vi "config_TRIG1.vi"(10 "VISA resource name":refnum<visa-resource-name>="TRIG") -> ()   [LabVIEW 2011]
uses:
  global.vi
  <vilib>/Platform/browser.llb/Open URL in Default Browser (string).vi
panel:
  out "delay array":dbl[](array[numeric])=[0.0, 4.7525e-05, 0.0, 5.65e-06, 0.0, 5.65e-06, 7.5e-06, 4.75e-05, 7.3e-06, 1.23e-05]
  in  "duration":dbl[](array[numeric])=[47.525000000000006, 5.65, 5.65, 40.0, 5.0] min=0.0 format="%.3f"
  in  "start time":dbl[](array[numeric])=[0.0, 0.0, 0.0, 7.5, 7.300000000000001] format="%.3f"
  in  "time unit":enum16{"s", "ms", "us", "ns"}(ring)=enum."us"
  in  "Reset TRIG":bool
  in  "write config":bool
  in  "stop":bool
  in  "help":bool
  out "update front panel":bool
  # "Configure Delay Generator (TRIG)"
  # "Polarity"
  # "NEGATIVE"
  # "POSITIVE"
  # "Nozzle"
  # "power AMP"
  # "AWG"
  # "SWITCH"
  # "OSC"
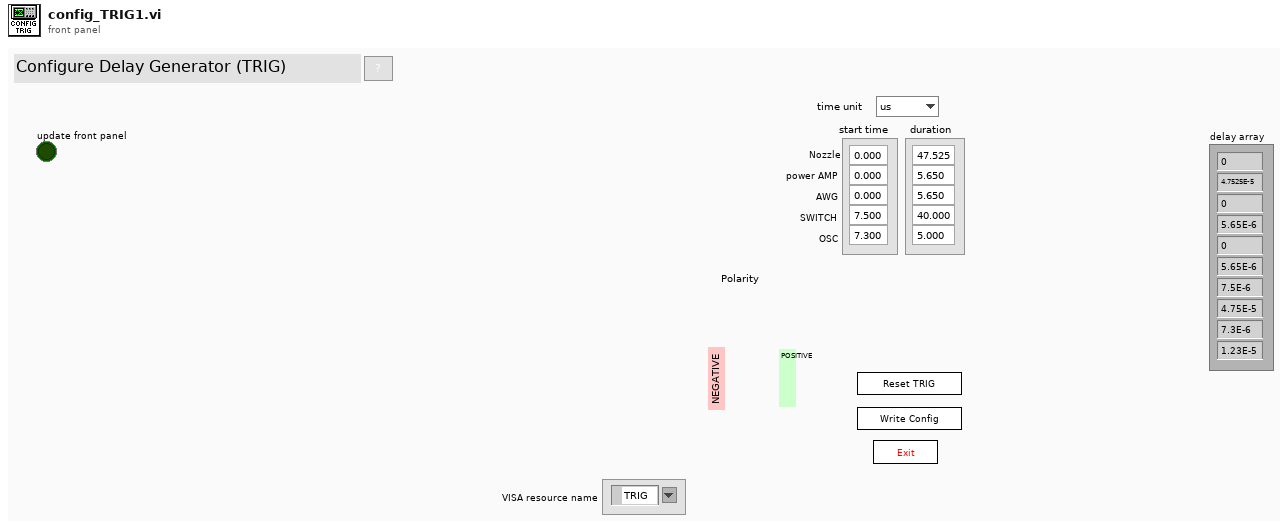
[diagram p1: front panel]
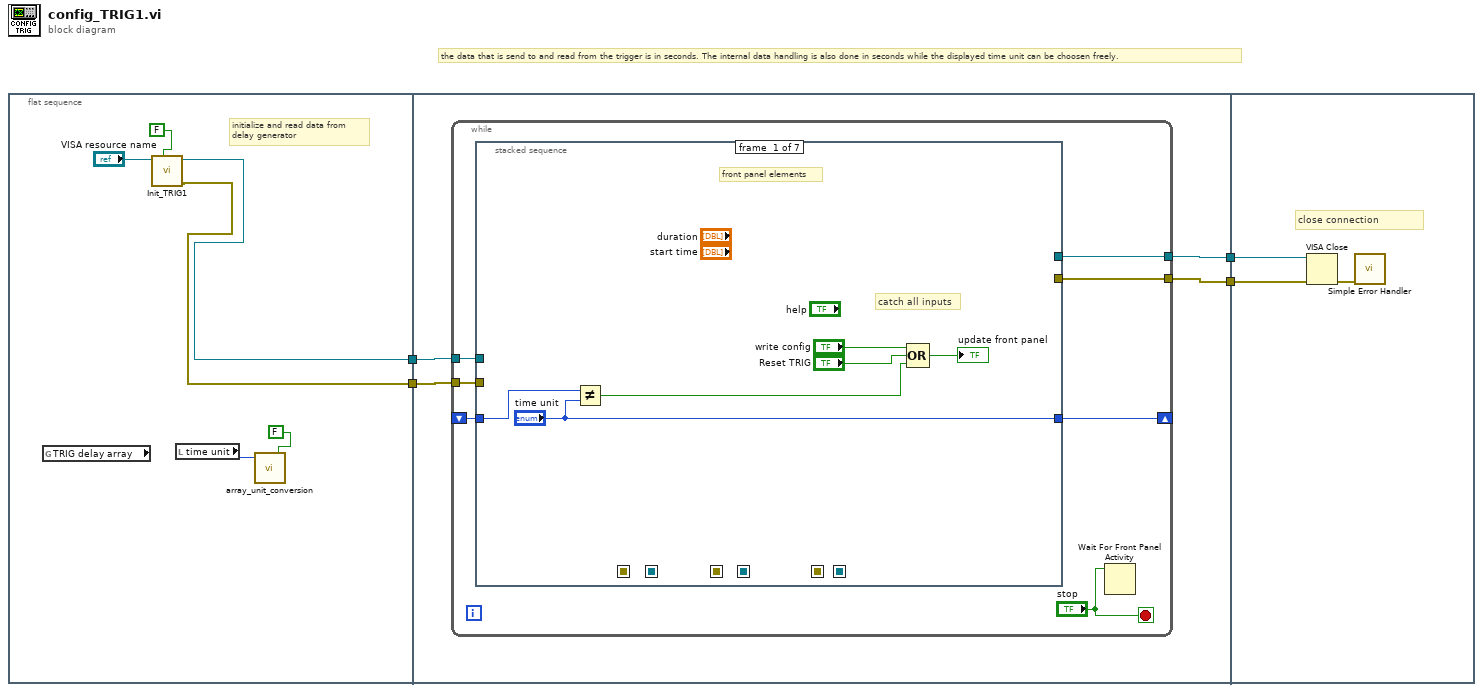
[diagram p0: block diagram]
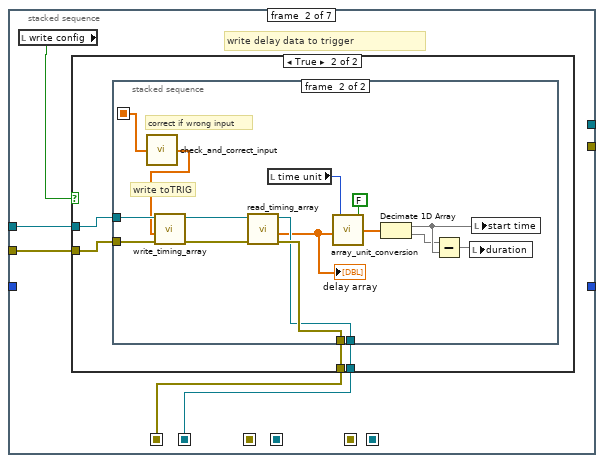
[diagram p2: hidden frame]
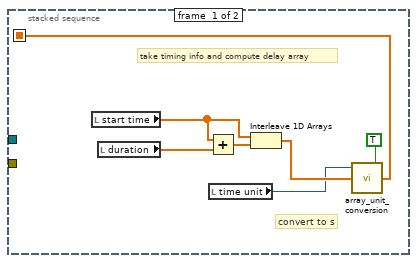
[diagram p4: hidden frame]
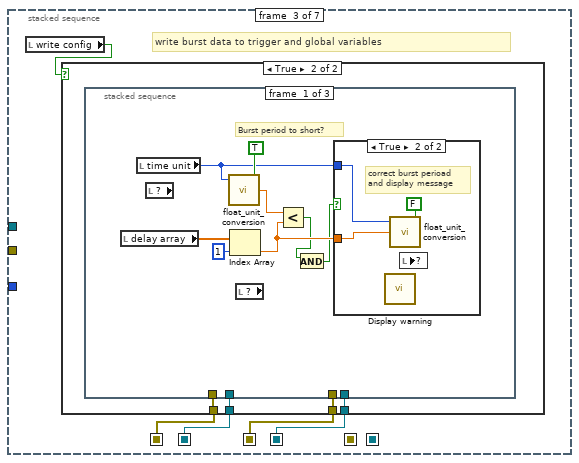
[diagram p5: hidden frame]
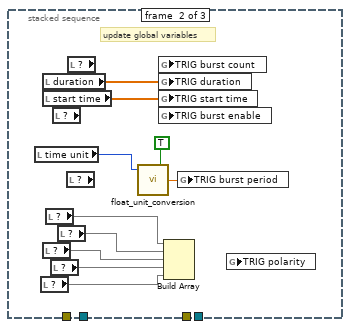
[diagram p8: hidden frame]
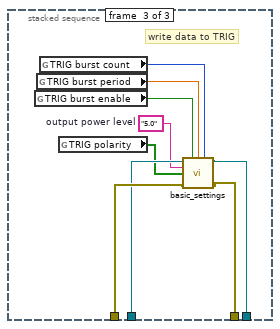
[diagram p9: hidden frame]
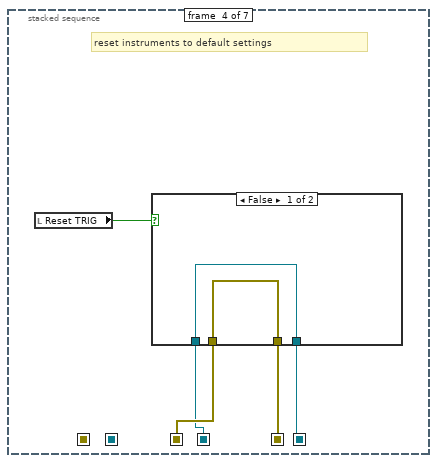
[diagram p10: hidden frame]
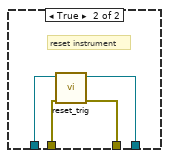
[diagram p11: hidden frame]
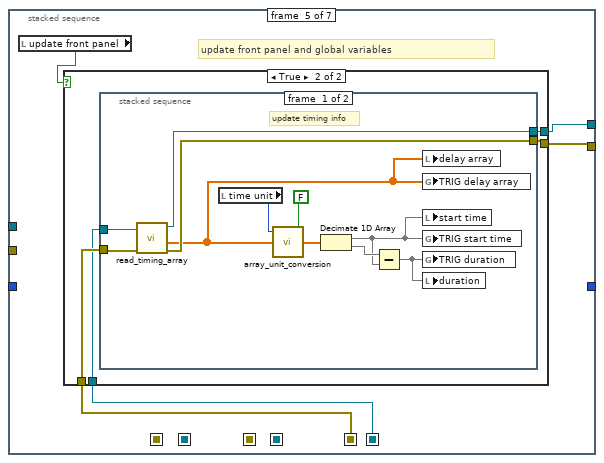
[diagram p12: hidden frame]
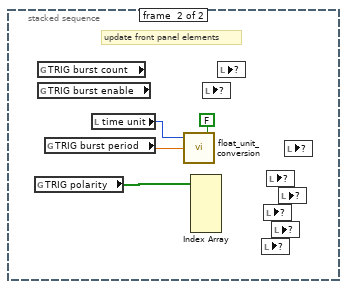
[diagram p14: hidden frame]
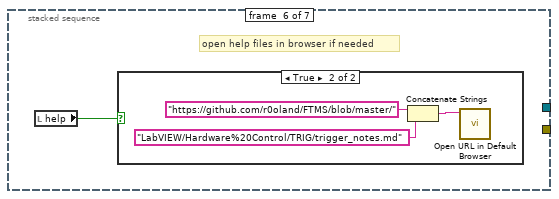
[diagram p15: hidden frame]
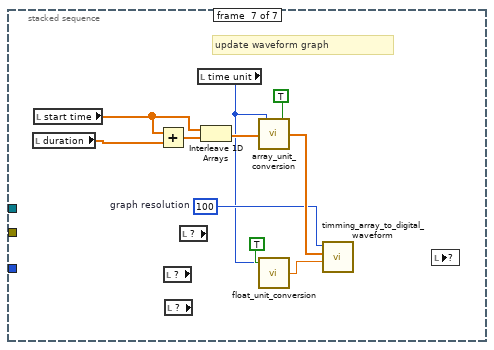
[diagram p17: hidden frame]
diagram:
  # "the data that is send to and read from the trigger is in seconds. The internal data handling is also done in seconds while the displayed time unit can be choosen freely."
  n1 = flat-sequence {
    tunnel: [w6] -> w4
    tunnel: [w5] -> w3
    tunnel: w4 -> [w14]
    tunnel: w3 -> [w13]
    tunnel: [w12] -> w2
    tunnel: [w11] -> w1
    tunnel: w2 -> [w155]
    tunnel: w1 -> [w154]
    frame #0 {
      # "initialize and read data from \ndelay generator"
      n2 = global read "global.vi" "TRIG delay array"() -> ()  [unwired: 1 out]
      n3 = call "Init_TRIG1.vi"("reset"=FALSE ("reset TRIG"), "VISA resource name"="VISA resource name") -> ("error out"=w5:errorcluster, "VISA resource name out"=w6:refnum<visa-resource-name>)  [unwired: 8 in]
      n4 = local read "time unit"() -> (w10:enum16{"s", "ms", "us", "ns"})
      n5 = call "array_unit_conversion.vi"("inverse function (arb. unit to s)?"=FALSE, "time unit"=w10) -> ()  [unwired: 3 in, 1 out]
    }
    frame #1 {
      n6 = while {
        tunnel: w13 -> [w19]
        tunnel: [w21] -> w12
        tunnel: [w20] -> w11
        tunnel: w14 -> [w17]
        shift-right: [w16] -> _
        shift-left: _ -> [w15]
        stop <- "stop" stop-if-true
        n7 = stacked-sequence {
          seq-local: [_ w28 _ _ _ _ _] -> [_ _ w64 _ _ _ _]
          seq-local: [_ w29 _ _ _ _ _] -> [_ _ w61 _ _ _ _]
          seq-local: [_ _ w62 _ _ _ _] -> [_ _ _ w106 _ _ _]
          seq-local: [_ _ w63 _ _ _ _] -> [_ _ _ w105 _ _ _]
          seq-local: [_ _ _ w102 _ _ _] -> [_ _ _ _ w116 _ _]
          seq-local: [_ _ _ w103 _ _ _] -> [_ _ _ _ w115 _ _]
          tunnel: w17 -> [_ w31 _ _ _ _ _]
          tunnel: w19 -> [_ w30 _ _ _ _ _]
          tunnel: [_ _ _ _ w114 _ _] -> w20
          tunnel: [_ _ _ _ w117 _ _] -> w21
          tunnel: ["time unit" _ _ _ _ _ _] -> w16
          tunnel: w15 -> [w25 _ _ _ _ _ _]
          frame #0 {
            # "front panel elements"
            # "catch all inputs"
            n8 = Not Equal?(x=w25, y="time unit") -> (x != y?=w22:bool)
            n9 = Compound Arithmetic op=OR("write config", "Reset TRIG", w22) -> (→"update front panel":bool)
          }
          frame #1 {
            # "write delay data to trigger"
            n10 = local read "write config"() -> (w32:bool)
            n11 = case shown="True" w32 {
              tunnel: w31 -> [w34 w38]
              tunnel: w30 -> [w33 w37]
              tunnel: [w34 w36] -> w29
              tunnel: [w33 w35] -> w28
              frame False {
              }
              frame True {
                n12 = stacked-sequence {
                  seq-local: [w41 _] -> [_ w56]
                  tunnel: w38 -> [_ w60]
                  tunnel: w37 -> [_ w59]
                  tunnel: [_ w53] -> w36
                  tunnel: [_ w54] -> w35
                  frame #0 {
                    # "convert to s"
                    # "take timing info and compute delay array"
                    n13 = local read "start time"() -> (w40:dbl[])
                    n14 = local read "duration"() -> (w39:dbl[])
                    n15 = Add(x=w40, y=w39) -> (x+y=w45:dbl[])
                    n16 = local read "time unit"() -> (w42:enum16{"s", "ms", "us", "ns"})
                    n17 = Interleave 1D Arrays(w40, w45) -> (w43:dbl[])
                    n18 = call "array_unit_conversion.vi"("inverse function (arb. unit to s)?"=TRUE, "delay array"=w43, "time unit"=w42) -> ("output"=w41:dbl[])  [unwired: 2 in]
                  }
                  frame #1 {
                    # "write toTRIG"
                    # "correct if wrong input"
                    n19 = call "check_and_correct_input.vi"("delay array"=w56) -> ("corrrected delay array"=w55:dbl[])  [unwired: 4 in]
                    n20 = call "write_timing_array.vi"("error in"=w59, "delay array"=w55, "VISA resource in"=w60) -> ("error out 2"=w57:errorcluster, "VISA resource out"=w58:refnum<visa-resource-name>)  [unwired: 3 in]
                    n21 = call "read_timing_array.vi"("error in"=w57, "VISA resource in"=w58) -> ("error out 2"=w54:errorcluster, "delay array"=w46:dbl[], "VISA resource out"=w53:refnum<visa-resource-name>)  [unwired: 3 in]
                    "delay array" <- w46
                    n22 = local read "time unit"() -> (w48:enum16{"s", "ms", "us", "ns"})
                    n23 = call "array_unit_conversion.vi"("inverse function (arb. unit to s)?"=FALSE, "delay array"=w46, "time unit"=w48) -> ("output"=w50:dbl[])  [unwired: 2 in]
                    n24 = Decimate 1D Array(w50) -> (w51:dbl[], w47:dbl[])
                    n25 = Subtract(x=w47, y=w51) -> (x-y=w52:dbl[])
                    n26 = local write "duration"(w52) -> ()
                    n27 = local write "start time"(w51) -> ()
                  }
                }
              }
            }
          }
          frame #2 {
            # "write burst data to trigger and global variables"
            n28 = local read "write config"() -> (w65:bool)
            n29 = case shown="True" w65 {
              tunnel: w64 -> [w66 w69]
              tunnel: w61 -> [w67 w68]
              tunnel: [w67 w71] -> w63
              tunnel: [w66 w70] -> w62
              frame False {
              }
              frame True {
                n30 = stacked-sequence {
                  tunnel: [_ _ w101] -> w71
                  tunnel: [_ _ w100] -> w70
                  tunnel: w69 -> [_ _ w99]
                  tunnel: w68 -> [_ _ w98]
                  frame #0 {
                    # "Burst period to short?"
                    n31 = local read "delay array"() -> (w75:dbl[])
                    n32 = local read "time unit"() -> (w76:enum16{"s", "ms", "us", "ns"})
                    n33 = local read item#-1() -> ()  [unwired: 1 out]
                    n34 = call "float_unit_conversion.vi"("inverse function (arb. unit to s)?"=TRUE, "time unit"=w76) -> ("converted time"=w77:dbl)  [unwired: 3 in]
                    n35 = Index Array(array=w75, index=1) -> (element=w74:dbl)
                    n36 = local read item#-1() -> ()  [unwired: 1 out]
                    n37 = Less?(x=w77, y=w74) -> (x < y?=w73:bool)
                    n38 = And(x=w73) -> (x .and. y?=w72:bool)  [unwired: 1 in]
                    n39 = case shown="True" w72 {
                      tunnel: w76 -> [_ w81]
                      tunnel: w74 -> [_ w80]
                      frame False {
                      }
                      frame True {
                        # "correct burst perioad\nand display message"
                        n40 = call "Display warning"() -> ()  [unwired: 10 in, 2 out]
                        n41 = call "float_unit_conversion.vi"("inverse function (arb. unit to s)?"=FALSE, "time"=w80, "time unit"=w81) -> ()  [unwired: 2 in, 1 out]
                        n42 = local read item#-1() -> ()  [unwired: 1 in]
                      }
                    }
                  }
                  frame #1 {
                    # "update global variables"
                    n43 = local read "time unit"() -> (w83:enum16{"s", "ms", "us", "ns"})
                    n44 = local read item#-1() -> (w88)
                    n45 = local read "duration"() -> (w91:dbl[])
                    n46 = local read "start time"() -> (w92:dbl[])
                    n47 = local read item#-1() -> (w86)
                    n48 = local read item#-1() -> (w84)
                    n49 = local read item#-1() -> (w87)
                    n50 = local read item#-1() -> ()  [unwired: 1 out]
                    n51 = local read item#-1() -> (w85)
                    n52 = local read item#-1() -> ()  [unwired: 1 out]
                    n53 = local read item#-1() -> ()  [unwired: 1 out]
                    n54 = call "float_unit_conversion.vi"("inverse function (arb. unit to s)?"=TRUE, "time unit"=w83) -> ("converted time"=w89:dbl)  [unwired: 3 in]
                    n55 = global read "global.vi" "TRIG burst count"() -> ()  [unwired: 1 in]
                    n56 = global write "global.vi" "TRIG duration"(w91) -> ()
                    n57 = global write "global.vi" "TRIG start time"(w92) -> ()
                    n58 = global read "global.vi" "TRIG burst enable"() -> ()  [unwired: 1 in]
                    n59 = Build Array(w84, w85, w86, w87, w88) -> ()  [unwired: 1 out]
                    n60 = global write "global.vi" "TRIG burst period"(w89) -> ()
                    n61 = global read "global.vi" "TRIG polarity"() -> ()  [unwired: 1 in]
                  }
                  frame #2 {
                    w94 = "5.0"  # output power level
                    # "write data to TRIG"
                    n62 = global read "global.vi" "TRIG burst enable"() -> (w95:bool)
                    n63 = global read "global.vi" "TRIG burst period"() -> (w96:dbl)
                    n64 = global read "global.vi" "TRIG burst count"() -> (w97:i32)
                    n65 = global read "global.vi" "TRIG polarity"() -> (w93:bool[])
                    n66 = call "basic_settings.vi"("VISA resource name"=w98, "Burst enable?"=w95, "burst period (s)"=w96, "burst count"=w97, "power level"=w94, "polarity"=w93, "error in (no error)"=w99) -> ("VISA resource name out"=w101:refnum<visa-resource-name>, "error out"=w100:errorcluster)  [unwired: 7 in]
                  }
                }
              }
            }
          }
          frame #3 {
            # "reset instruments to default settings"
            n67 = local read "Reset TRIG"() -> (w104:bool)
            n68 = case shown="False" w104 {
              tunnel: w106 -> [w107 w112]
              tunnel: w105 -> [w108 w111]
              tunnel: [w108 w109] -> w103
              tunnel: [w107 w110] -> w102
              frame False {
              }
              frame True {
                # "reset instrument"
                n69 = call "reset_trig.vi"("error in (no error)"=w112, "VISA resource name"=w111) -> ("error out"=w110:errorcluster, "VISA resource name out"=w109:refnum<visa-resource-name>)  [unwired: 8 in]
              }
            }
          }
          frame #4 {
            # "update front panel and global variables"
            n70 = local read "update front panel"() -> (w113:bool)
            n71 = case shown="True" w113 {
              tunnel: [w119 w123] -> w117
              tunnel: [w118 w122] -> w114
              tunnel: w116 -> [w118 w121]
              tunnel: w115 -> [w119 w120]
              frame False {
              }
              frame True {
                n72 = stacked-sequence {
                  tunnel: [w134 _] -> w123
                  tunnel: [w133 _] -> w122
                  tunnel: w121 -> [w128 _]
                  tunnel: w120 -> [w127 _]
                  frame #0 {
                    # "update timing info"
                    n73 = call "read_timing_array.vi"("error in"=w128, "VISA resource in"=w127) -> ("error out 2"=w133:errorcluster, "delay array"=w124:dbl[], "VISA resource out"=w134:refnum<visa-resource-name>)  [unwired: 3 in]
                    n74 = local read "time unit"() -> (w131:enum16{"s", "ms", "us", "ns"})
                    n75 = call "array_unit_conversion.vi"("inverse function (arb. unit to s)?"=FALSE, "delay array"=w124, "time unit"=w131) -> ("output"=w129:dbl[])  [unwired: 2 in]
                    n76 = Decimate 1D Array(w129) -> (w126:dbl[], w132:dbl[])
                    n77 = Subtract(x=w132, y=w126) -> (x-y=w125:dbl[])
                    n78 = local write "delay array"(w124) -> ()
                    n79 = global write "global.vi" "TRIG delay array"(w124) -> ()
                    n80 = local write "start time"(w126) -> ()
                    n81 = global write "global.vi" "TRIG start time"(w126) -> ()
                    n82 = global write "global.vi" "TRIG duration"(w125) -> ()
                    n83 = local write "duration"(w125) -> ()
                  }
                  frame #1 {
                    # "update front panel elements"
                    n84 = global read "global.vi" "TRIG polarity"() -> (w138:bool[])
                    n85 = global read "global.vi" "TRIG burst count"() -> ()  [unwired: 1 out]
                    n86 = global read "global.vi" "TRIG burst enable"() -> ()  [unwired: 1 out]
                    n87 = global read "global.vi" "TRIG burst period"() -> (w136:dbl)
                    n88 = local read "time unit"() -> (w135:enum16{"s", "ms", "us", "ns"})
                    n89 = call "float_unit_conversion.vi"("inverse function (arb. unit to s)?"=FALSE, "time"=w136, "time unit"=w135) -> ()  [unwired: 2 in, 1 out]
                    n90 = Index Array(array=w138) -> ()  [unwired: 5 in, 5 out]
                    n91 = local read item#-1() -> ()  [unwired: 1 in]
                    n92 = local read item#-1() -> ()  [unwired: 1 in]
                    n93 = local read item#-1() -> ()  [unwired: 1 in]
                    n94 = local read item#-1() -> ()  [unwired: 1 in]
                    n95 = local read item#-1() -> ()  [unwired: 1 in]
                    n96 = local read item#-1() -> ()  [unwired: 1 in]
                    n97 = local read item#-1() -> ()  [unwired: 1 in]
                    n98 = local read item#-1() -> ()  [unwired: 1 in]
                  }
                }
              }
            }
          }
          frame #5 {
            # "open help files in browser if needed"
            n99 = local read "help"() -> (w139:bool)
            n100 = case shown="True" w139 {
              frame False {
              }
              frame True {
                n101 = Concatenate Strings("https://github.com/r0oland/FTMS/blob/master/" ("string"), "LabVIEW/Hardware%20Control/TRIG/trigger_notes.md" ("string")) -> (w142:string)
                n102 = call-poly <vilib>:"Open URL in Default Browser.vi"("URL"=w142) -> ()  [unwired: 5 in, 2 out]
              }
            }
          }
          frame #6 {
            w148 = 100  # graph resolution
            # "update waveform graph"
            n103 = local read "duration"() -> (w146:dbl[])
            n104 = local read "start time"() -> (w147:dbl[])
            n105 = Add(x=w147, y=w146) -> (x+y=w152:dbl[])
            n106 = local read item#-1() -> ()  [unwired: 1 out]
            n107 = local read item#-1() -> ()  [unwired: 1 out]
            n108 = local read item#-1() -> ()  [unwired: 1 out]
            n109 = local read "time unit"() -> (w144:enum16{"s", "ms", "us", "ns"})
            n110 = Interleave 1D Arrays(w147, w152) -> (w150:dbl[])
            n111 = call "array_unit_conversion.vi"("inverse function (arb. unit to s)?"=TRUE, "delay array"=w150, "time unit"=w144) -> ("output"=w149:dbl[])  [unwired: 2 in]
            n112 = call "float_unit_conversion.vi"("inverse function (arb. unit to s)?"=TRUE, "time unit"=w144) -> ("converted time"=w143:dbl)  [unwired: 3 in]
            n113 = call "timming_array_to_digital_waveform.vi"("resolution"=w148, "delay array"=w149, "burst period"=w143) -> ()  [unwired: 3 in, 2 out]
            n114 = local read item#-1() -> ()  [unwired: 1 in]
          }
        }
        n115 = Wait For Front Panel Activity(3:"stop") -> ()  [unwired: 2 in, 1 out]
      }
    }
    frame #2 {
      # "close connection"
      n116 = VISA Close(VISA resource name=w155, error in (no error)=w154) -> (error out=w153:errorcluster)
      n117 = call <vilib>:"Simple Error Handler.vi"("error in (no error)"=w153) -> ()  [unwired: 4 in, 5 out]
    }
  }
